vi "addNode.vi"(0 "reference":refnum<class "Graph.lvclass">, 1 "node":refnum<class "AbstractNode.lvclass">, 2 "point":T1 {"y" format="%.2f"; "x" format="%.2f"}, 5 "error in (no error)":errorcluster) -> (14 "reference out":refnum<class "Graph.lvclass">, 19 "error out":errorcluster)   [LabVIEW 2012, in "Graph.lvclass"]
doc: "public void addNode(Node n, Point2D p)"
uses:
  <resource>/Framework/Providers/Open_GDS/UML/Graph_class/Graph.lvclass
  <resource>/Framework/Providers/Open_GDS/UML/AbstractNode_class/AbstractNode.lvclass
  <resource>/Framework/Providers/Open_GDS/UML/General/Point/Point Point2D.ctl
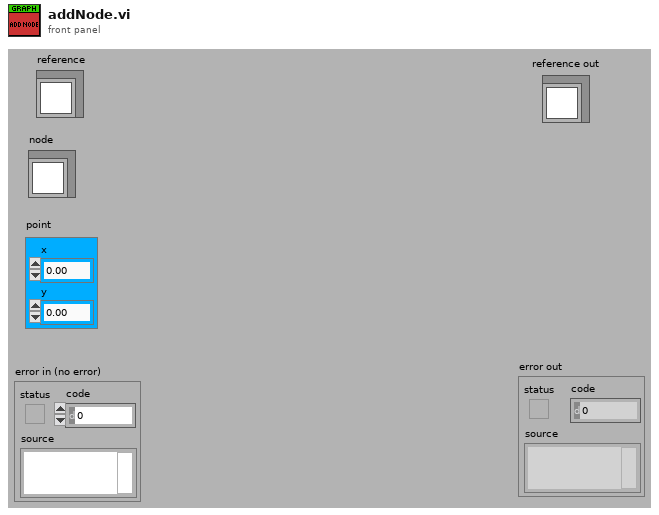
[diagram p1: front panel]
types:
  T1 = typedef "Point Point2D.ctl" = cluster{"x":dbl, "y":dbl}
  T2 = typedef "Rectangle Rectangle2D.ctl" = cluster{"x":dbl, "y":dbl, "width":dbl, "height":dbl}
  T3 = typedef "Graph.lvclass/ObjectAttributes.ctl" = cluster{"nodes":refnum<class "AbstractNode.lvclass">[], "edges":refnum<class "AbstractEdge.lvclass">[], "nodesToBeRemoved":refnum<class "AbstractNode.lvclass">[], "edgesToBeRemoved":refnum<class "AbstractEdge.lvclass">[], "needsLayout":bool, "LayoutNodes":refnum<class "AbstractNode.lvclass">[]}
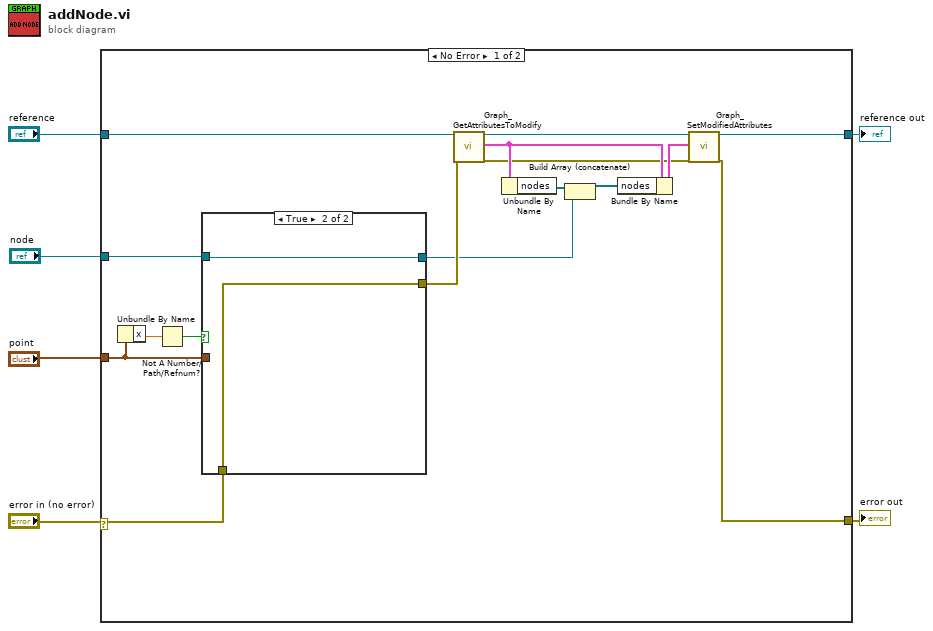
[diagram p0: block diagram]
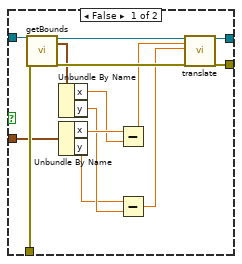
[diagram p2: hidden frame]
diagram:
  n1 = case shown="No Error" "error in (no error)" {
    selector: "error in (no error)" -> [w19 w39]
    tunnel: "reference" -> [w22 w40]
    tunnel: [w21 w39] -> w5
    tunnel: [w20 w40] -> w4
    tunnel: "node" -> [w18 _]
    tunnel: "point" -> [w9 _]
    frame No Error {
      n2 = Unbundle By Name(w9) -> ("x"=w8:dbl)
      n3 = Not A Number/Path/Refnum?(number/path/refnum=w8) -> (NaN/Path/Refnum?=w7:bool)
      n4 = case shown="True" w7 {
        tunnel: w19 -> [w36 w37]
        tunnel: w18 -> [w35 w38]
        tunnel: w9 -> [w34 _]
        tunnel: [w32 w37] -> w11
        tunnel: [w30 w38] -> w10
        frame False {
          n5 = call-dynamic "getBounds.vi"("reference"=w35, "error in (no error)"=w36) -> ("reference out"=w31:refnum<class "AbstractNode.lvclass">, "bounds"=w29:T2, "error out"=w33:errorcluster)  [unwired: 15 in]
          n6 = Unbundle By Name(w29) -> ("x"=w27:dbl, "y"=w26:dbl)
          n7 = Unbundle By Name(w34) -> ("x"=w28:dbl, "y"=w25:dbl)
          n8 = Subtract(x=w28, y=w27) -> (x-y=w23:dbl)
          n9 = Subtract(x=w25, y=w26) -> (x-y=w24:dbl)
          n10 = call-dynamic "translate.vi"("reference"=w31, "dx"=w23, "dy"=w24, "error in (no error)"=w33) -> ("reference out"=w30:refnum<class "AbstractNode.lvclass">, "error out"=w32:errorcluster)  [unwired: 14 in]
        }
        frame True {
        }
      }
      n11 = call <resource>:"Graph_GetAttributesToModify.vi"("reference in"=w22, "error in (no error)"=w11) -> ("reference out"=w17:refnum<class "Graph.lvclass">, "Attributes"=w15:T3, "error out"=w14:errorcluster)  [unwired: 1 in, 14 out]
      n12 = Unbundle By Name(w15) -> ("nodes"=w13:refnum<class "AbstractNode.lvclass">[])
      n13 = Build Array (concatenate)(w13, w10) -> (w12:refnum<class "AbstractNode.lvclass">[])
      n14 = Bundle By Name(cluster=w15, "nodes"=w12) -> (w16:T3)
      n15 = call <resource>:"Graph_SetModifiedAttributes.vi"("reference in"=w17, "Attributes"=w16, "error in (no error)"=w14) -> ("reference out"=w20:refnum<class "Graph.lvclass">, "error out"=w21:errorcluster)  [unwired: 3 in, 12 out]
    }
    frame Error {
    }
  }
  "reference out" <- w4
  "error out" <- w5
